vi "Choose Next XNET Interface Value.vi"(8 "error in":errorcluster, 11 "Databases section Ref":T1 format="%.0x") -> (0 "error out":errorcluster, 2 "Next Available Value":u16, 3 "Databases section Ref out":T1 format="%.0x")   [LabVIEW 2020, in "Communication Bus Template System Explorer.lvlib" / "Implementation.lvlib"]
uses:
  Implementation.lvlib
  <vilib>/NI VeriStand/Custom Device Tools/Custom Device Utility Library/Custom Device Utility Library.lvlib
  Scripting/Constants.vi
  Scripting/Communication Bus Template Scripting.lvlib
  <vilib>/NI VeriStand/Custom Device Tools/Custom Device Utility Library/NI VeriStand - Search for All Items by GUID.vi
  <vilib>/NI VeriStand/Custom Device API/Custom Device Item Ref.ctl
  <vilib>/NI VeriStand/Custom Device API/Custom Device API.lvlib
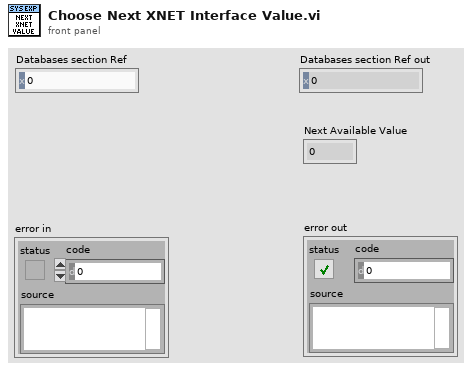
[diagram p1: front panel]
types:
  T1 = typedef "Custom Device API.lvlib/Custom Device Item Ref.ctl" = u64
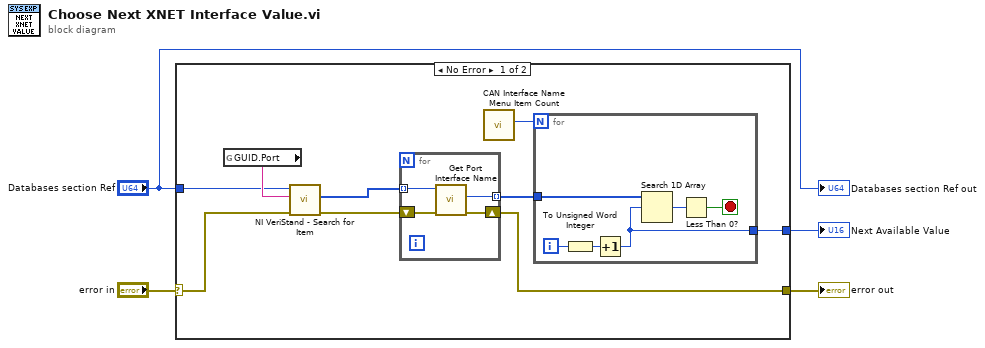
[diagram p0: block diagram]
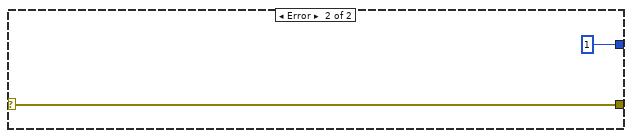
[diagram p2: hidden frame]
diagram:
  n1 = case shown="No Error" "error in" {
    selector: "error in" -> [w6 w25]
    tunnel: [w5 w25] -> w3
    tunnel: "Databases section Ref" -> [w12 _]
    tunnel: [w7 u16 1] -> w2
    frame No Error {
      n2 = global read "Constants.vi" "GUID.Port"() -> (w13:string)
      n3 = call-poly <vilib>:"NI VeriStand - Search for Item.vi"("error in"=w6, "Item GUID"=w13, "Section Ref in"=w12) -> ("error out"=w11:errorcluster, "Item Refs"=w9:T1[])  [unwired: 5 in, 2 out]
      n4 = for {
        tunnel: w9 -> [w16] mode=indexing
        tunnel: [w15] -> w8 mode=indexing
        shift-right: [w14] -> w5
        shift-left: w11 -> [w17]
        n5 = call "Get Port Interface Name.vi"("error in"=w17, "Port Ref"=w16) -> ("error out"=w14:errorcluster, "CAN Interface Number"=w15:u16)  [unwired: 6 in, 2 out]
      }
      n6 = call "CAN Interface Name Menu Item Count.vi"() -> ("number of menu items"=w10:u16)  [unwired: 11 in]
      n7 = for {
        N: w10 -> [_]
        tunnel: w8 -> [w23]
        tunnel: [w18] -> w7
        i -> [w22]
        stop <- w19 stop-if-true
        n8 = To Unsigned Word Integer(number=w22) -> (unsigned 16bit integer=w21:u16)
        n9 = Increment(x=w21) -> (x+1=w18:u16)
        n10 = Search 1D Array(1D array=w23, element=w18) -> (index of element=w20:i32)  [unwired: 1 in]
        n11 = Less Than 0?(x=w20) -> (x < 0?=w19:bool)
      }
    }
    frame Error {
    }
  }
  "error out" <- w3
  "Next Available Value" <- w2
  "Databases section Ref out" <- "Databases section Ref"
